vi "TestPVCam.vi"() -> ()   [LabVIEW 2023, in "Photometrics Camera.lvlib"]
uses:
  Photometrics Camera.lvlib
  Resources/Type Defs/Camera Settings.ctl
  Resources/Type Defs/Physical Camera Assignment.ctl
  Photometrics Camera.lvclass
  Camera Messages/Start Live Mode Msg/Start Live Mode Msg.lvclass/Start Live Mode Msg.ctl
  <vilib>/ActorFramework/Message Enqueuer/Message Enqueuer.lvclass/Message Enqueuer.ctl
  <vilib>/ActorFramework/Message Enqueuer/Enqueue.vi
  Camera Messages/Start Live Mode Msg/Start Live Mode Msg.lvclass
  Camera Messages/Stop Live Mode Msg/Stop Live Mode Msg.lvclass
  <vilib>/ActorFramework/Stop Msg/Stop Msg.lvclass
  <vilib>/ActorFramework/Message Priority Queue/Priority Enqueue.vi
  <vilib>/ActorFramework/Actor/Actor.lvclass
panel:
  in  "Physical Camera Assignment":T1[](array[typedef])=[{"Channel Name"="Cy3", "Serial Number"="A24D723024", "Flip Vertically"=FALSE, "Flip Horizontally"=FALSE, "photonsPerCount"=0.5, "wavelength"=532}, {"Channel Name"="Cy5", "Serial Number"="A24C723032", "Flip Vertically"=FALSE, "Flip Horizontally"=FALSE, "photonsPerCount"=0.5, "wavelength"=640}]
  in  "stop":bool
  in  "Camera Settings":T2={"Exposure Time (ms)"=100.0, "Binning"=enum."2x2", "Scan Mode"=-1, "Frames to Acquire"=1000.0, "Pixel Correction"=FALSE, "Frames to Skip"=0, "File Path"=path "", "Duty cycle"=1.0, "ALEX"=FALSE, "Shutter Enable"=[], "fluidics trigger frame"=0, "Bit Depth"=0, "Image Width (px)"=0, "Image Height (px)"=0, "Horizontal Offset (px)"=0, "Vertical Offset (px)"=0} {"fluidics trigger frame" max=60000 step=1; "Exposure Time (ms)" min=1.0 max=10000.0 step=1.0}
  out "error out":errorcluster
  in  "error in (no error)":errorcluster
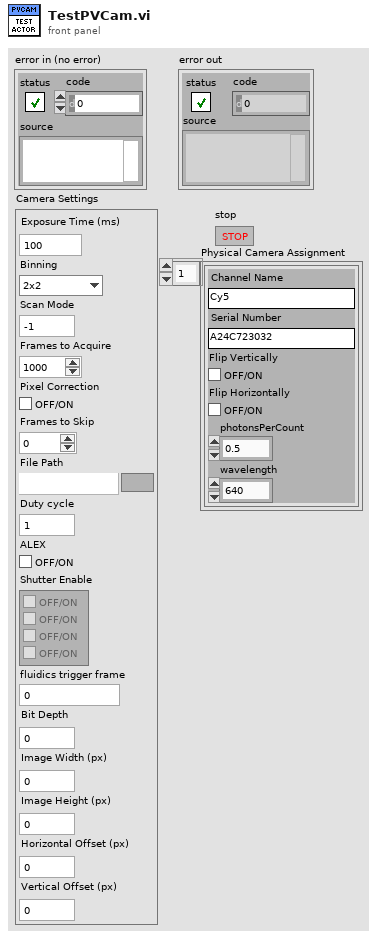
[diagram p1: front panel]
types:
  T1 = typedef "Physical Camera Assignment.ctl" = cluster{"Channel Name":string, "Serial Number":string, "Flip Vertically":bool, "Flip Horizontally":bool, "photonsPerCount":dbl, "wavelength":i16}
  T2 = typedef "Camera Settings.ctl" = cluster{"Exposure Time (ms)":dbl, "Binning":enum16{"1x1", "2x2", "4x4"}, "Scan Mode":i32, "Frames to Acquire":dbl, "Pixel Correction":bool, "Frames to Skip":u32, "File Path":path, "Duty cycle":dbl, "ALEX":bool, "Shutter Enable":bool[], "fluidics trigger frame":u16, "Bit Depth":u16, "Image Width (px)":u16, "Image Height (px)":u16, "Horizontal Offset (px)":u16, "Vertical Offset (px)":u16}
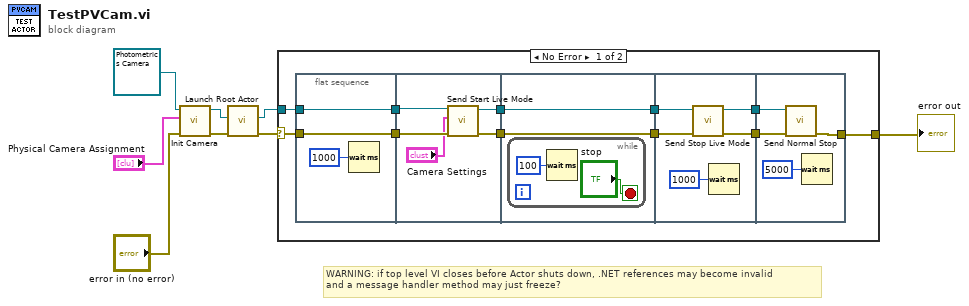
[diagram p0: block diagram]
diagram:
  # "WARNING: if top level VI closes before Actor shuts down, .NET references may become invalid\nand a message handler method may just freeze?"
  n1 = call-dynamic "Init Camera.vi"("error in (no error)"="error in (no error)", "Physical Camera Assignment"="Physical Camera Assignment", "Photometrics Camera in"=refnum<class "Photometrics Camera.lvclass"> refnum ("Photometrics Camera.lvlib:Photometrics Camera.lvclass")) -> ("error out"=w7:errorcluster, "Photometrics Camera out"=w4:refnum<class "Photometrics Camera.lvclass">)  [unwired: 7 in]
  n2 = call <vilib>:"Launch Root Actor.vi"("error in (no error)"=w7, "Actor"=w4) -> ("error out"=w1:errorcluster, "Actor's Enqueuer"=w8:refnum<class "Message Enqueuer.lvclass">)  [unwired: 8 in]
  n3 = case shown="No Error" w1 {
    selector: w1 -> [w9 w41]
    tunnel: w8 -> [w11 _]
    tunnel: [w10 w41] -> w2
    frame No Error {
      n4 = flat-sequence {
        tunnel: w11 -> [w22]
        tunnel: w9 -> [w20]
        tunnel: [w22] -> w19
        tunnel: [w20] -> w18
        tunnel: w19 -> [w25]
        tunnel: w18 -> [w27]
        tunnel: [w26] -> w17
        tunnel: [w23] -> w16
        tunnel: [w29] -> w15
        tunnel: [w28] -> w14
        tunnel: w17 -> [w29]
        tunnel: w16 -> [w28]
        tunnel: w15 -> [w35]
        tunnel: w14 -> [w34]
        tunnel: [w32] -> w13
        tunnel: [w33] -> w12
        tunnel: w13 -> [w39]
        tunnel: w12 -> [w40]
        tunnel: [w38] -> w10
        frame #0 {
          n5 = Wait (ms)(milliseconds to wait=u32 1000) -> ()  [unwired: 1 out]
        }
        frame #1 {
          n6 = call "Send Start Live Mode.vi"("error in (no error)"=w27, "Camera Settings"="Camera Settings", "Message Enqueuer"=w25) -> ("error out"=w23:errorcluster, "Message Enqueuer out"=w26:refnum<class "Message Enqueuer.lvclass">)  [unwired: 7 in]
        }
        frame #2 {
          n7 = while {
            stop <- "stop" stop-if-true
            n8 = Wait (ms)(milliseconds to wait=u32 100) -> ()  [unwired: 1 out]
          }
        }
        frame #3 {
          n9 = call "Send Stop Live Mode.vi"("error in (no error)"=w34, "Message Enqueuer"=w35) -> ("error out"=w33:errorcluster, "Message Enqueuer out"=w32:refnum<class "Message Enqueuer.lvclass">)  [unwired: 8 in]
          n10 = Wait (ms)(milliseconds to wait=u32 1000) -> ()  [unwired: 1 out]
        }
        frame #4 {
          n11 = call <vilib>:"Send Normal Stop.vi"("error in (no error)"=w40, "Message Enqueuer"=w39) -> ("error out"=w38:errorcluster)  [unwired: 9 in]
          n12 = Wait (ms)(milliseconds to wait=u32 5000) -> ()  [unwired: 1 out]
        }
      }
    }
    frame Error {
    }
  }
  "error out" <- w2
